vi "Multiple test points on oscilliscope.vi"(11 "VISA resource name":refnum<visa-resource-name>="USB0::0x1AB1::0x0488::DS1BA202100064::INSTR") -> ()   [LabVIEW 2018]
uses:
  <instrlib>/RIGOL DS1000 Series/Public/Data/Read (Single Waveform).vi
  <instrlib>/RIGOL DS1000 Series/RIGOL DS1000 Series.lvlib
panel:
  out "Waveform Data":waveform(dbl)(graph)
  in  "Measurement Function (0: Voltage Vpp) 2":u16(ring) items=["Voltage Vpp", "Voltage Max", "Voltage Min", "Amplitude", "Voltage TOP", "Voltage Base", "Voltage Average", "Voltage RMS", "Overshoot", "Preshoot", "Frequency", "Rise Time", "Fall Time", "Period", "Positive Width", "Negative Width", "Positive Duty", "Negative Duty"]
  out "Measured Value 2":dbl
  in  "Measurement Function (0: Voltage Vpp)":u16(ring) items=["Voltage Vpp", "Voltage Max", "Voltage Min", "Amplitude", "Voltage TOP", "Voltage Base", "Voltage Average", "Voltage RMS", "Overshoot", "Preshoot", "Frequency", "Rise Time", "Fall Time", "Period", "Positive Width", "Negative Width", "Positive Duty", "Negative Duty"]
  out "Measured Value":dbl
  in  "Channel (0: Channel 1)":u16(ring) items=["Channel 1", "Channel 2", "Channel 3", "Channel 4"]
  in  "Stop":bool
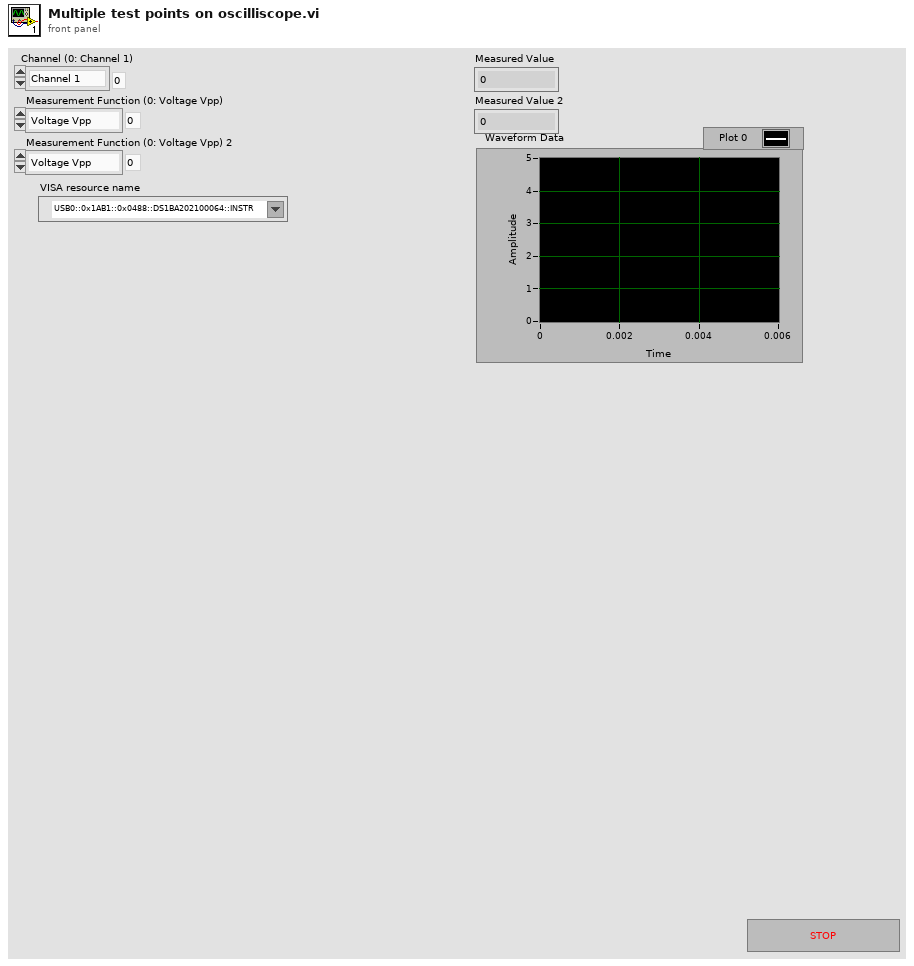
[diagram p1: front panel]
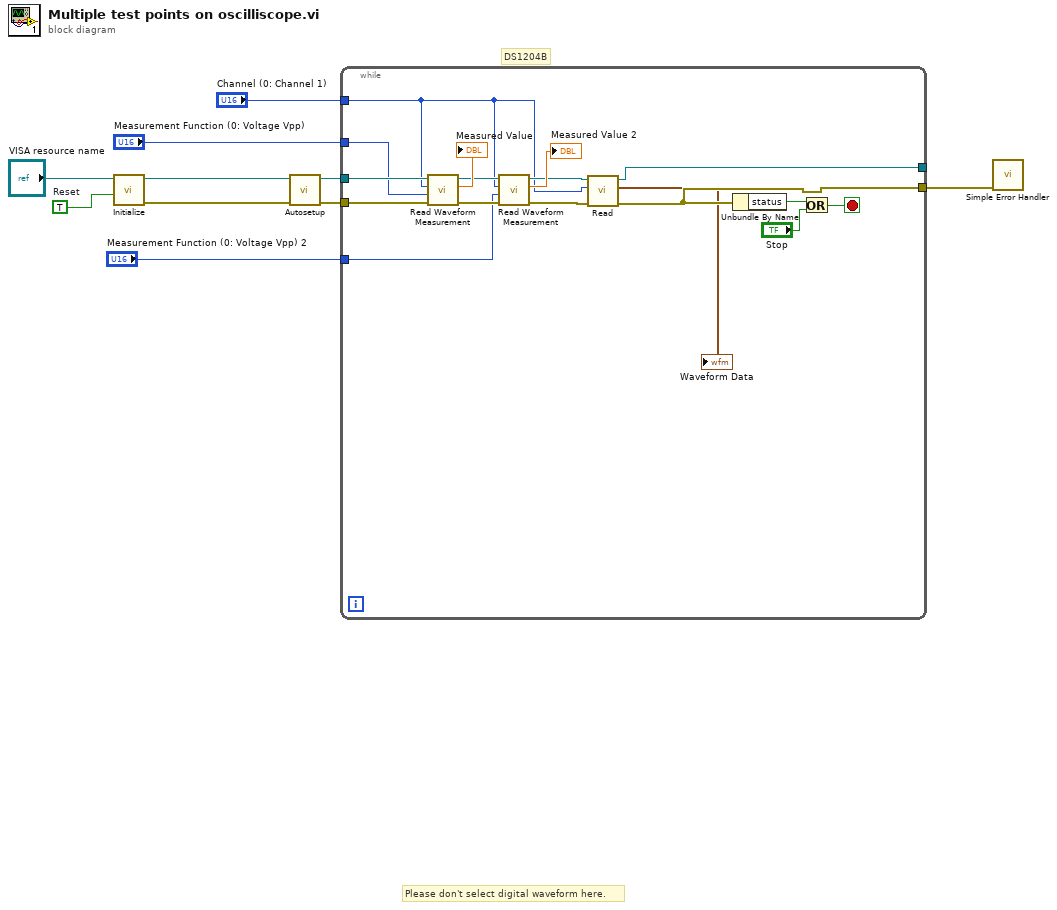
[diagram p0: block diagram]
diagram:
  w8 = TRUE  # Reset
  # "DS1204B"
  # "Please don't select digital waveform here."
  n1 = call <instrlib>:"Initialize.vi"("Reset (True)"=w8, "VISA resource name"="VISA resource name") -> ("error out"=w6:errorcluster, "VISA resource name out"=w7:refnum<visa-resource-name>)  [unwired: 2 in, 6 out]
  n2 = call <instrlib>:"Autosetup.vi"("error in (no error)"=w6, "VISA resource name"=w7) -> ("error out"=w9:errorcluster, "VISA resource name out"=w10:refnum<visa-resource-name>)  [unwired: 8 in]
  n3 = while {
    tunnel: w10 -> [w27]
    tunnel: w9 -> [w26]
    tunnel: [w14] -> w5
    tunnel: "Channel (0: Channel 1)" -> [w11]
    tunnel: "Measurement Function (0: Voltage Vpp)" -> [w21]
    tunnel: "Measurement Function (0: Voltage Vpp) 2" -> [w17]
    tunnel: [w15] -> _
    stop <- w25 stop-if-true
    n4 = call <instrlib>:"Read Waveform Measurement.vi"("error in (no error)"=w26, "Measurement Function (0: Voltage Vpp)"=w21, "Source (0: Channel 1)"=w11, "VISA resource name"=w27) -> ("error out"=w20:errorcluster, "Measured Value"=→"Measured Value":dbl, "VISA resource name out"=w19:refnum<visa-resource-name>)  [unwired: 5 in]
    n5 = call <instrlib>:"Read Waveform Measurement.vi"("error in (no error)"=w20, "Measurement Function (0: Voltage Vpp)"=w17, "Source (0: Channel 1)"=w11, "VISA resource name"=w19) -> ("error out"=w13:errorcluster, "Measured Value"=→"Measured Value 2":dbl, "VISA resource name out"=w16:refnum<visa-resource-name>)  [unwired: 5 in]
    n6 = call-poly <instrlib>:"Read.vi"("error in (no error)"=w13, "Channel (0: Channel 1)"=w11, "VISA resource name"=w16) -> ("error out"=w14:errorcluster, "Waveform Data"=→"Waveform Data":waveform(dbl), "VISA resource name out"=w15:refnum<visa-resource-name>)  [unwired: 6 in]
    n7 = Unbundle By Name(w14) -> ("status"=w24:bool)
    n8 = Or(x=w24, y="Stop") -> (x .or. y?=w25:bool)
  }
  n9 = call <vilib>:"Simple Error Handler.vi"("error in (no error)"=w5) -> ()  [unwired: 1 in, 8 out]
